vi "LaunchGUI.vi"(6 "Array":refnum<vi>[](array[refnum]), 10 "CtlRef":refnum<vi>, 11 "User Event in":refnum<user-event>) -> ()   [LabVIEW 2013]
uses:
  Controls/eventtypdef1.ctl
  Controls/controlFGV_TYPDEF.ctl
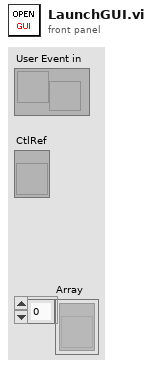
[diagram p1: front panel]
types:
  T1 = typedef "controlFGV_TYPDEF.ctl" = enum16{"read", "write", "clear"}
  T2 = typedef "eventtypdef1.ctl" = cluster{"label":string, "Sub Panel":refnum<vi>, "CtlRef":refnum<vi>, "This VI":refnum<vi>}
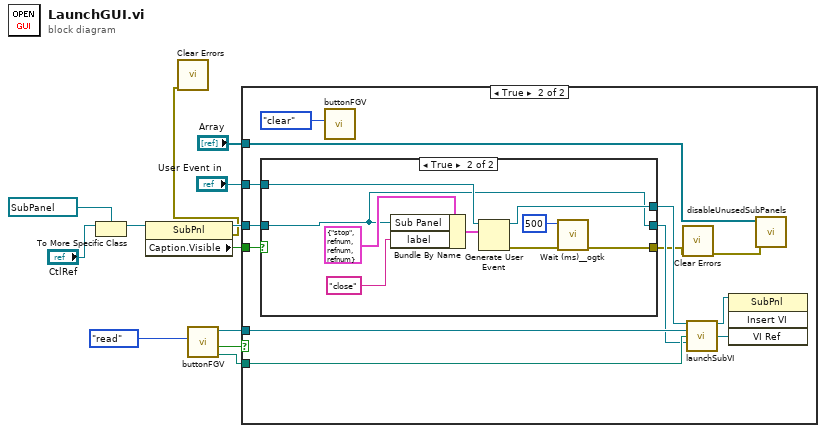
[diagram p0: block diagram]
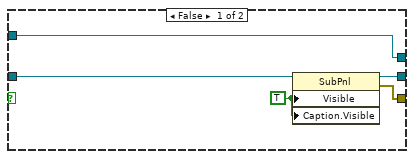
[diagram p3: hidden frame]
diagram:
  n1 = To More Specific Class(target class=refnum<vi> refnum ("Sub Panel"), reference="CtlRef") -> (specific class reference=w12:refnum<vi>)  [unwired: 1 in, 1 out]
  n2 = property class="SubPnl"(reference=w12) -> (reference out=w3:refnum<vi>, error out=w1:errorcluster, "Caption.Visible"=w8:bool)  [unwired: 1 in]
  n3 = call <vilib>:"Clear Errors.vi"("error in (no error)"=w1) -> ()  [unwired: 6 in, 1 out]
  n4 = call "buttonFGV.vi"("command"=controlFGV_TYPDEF."read") -> ("Path"=w6:path, "select subPanel"=w9:bool, "Boolean out"=w7:refnum<vi>)  [unwired: 8 in]
  n5 = case shown="True" w9 {
    tunnel: w6 -> [_ w25]
    tunnel: "User Event in" -> [_ w16]
    tunnel: w7 -> [_ w23]
    tunnel: "Array" -> [_ w24]
    tunnel: w8 -> [_ w17]
    tunnel: w3 -> [_ w22]
    frame False {
    }
    frame True {
      n6 = case shown="True" w17 {
        tunnel: [w29 w33] -> w14
        tunnel: w22 -> [w28 w36]
        tunnel: [w27 w36] -> w21
        tunnel: w16 -> [w26 w39]
        tunnel: [w26 w38] -> w15
        frame False {
          w30 = TRUE ("Visible")
          n7 = property class="SubPnl"(reference=w28, "Visible"=w30, "Caption.Visible"=w30) -> (reference out=w27:refnum<vi>, error out=w29:errorcluster)  [unwired: 1 in]
        }
        frame True {
          n8 = Bundle By Name(cluster=T2 {"label"="stop", "Sub Panel"=refnum, "CtlRef"=refnum, "This VI"=refnum} ("event data"), "Sub Panel"=w36, "label"="close") -> (w31:T2)
          n9 = Generate User Event(user event=w39, event data cluster=w31) -> (user event out=w38:refnum<user-event>, error out=w34:errorcluster)  [unwired: 2 in]
          n10 = call <userlib>:"Wait (ms)__ogtk.vi"("error in (no error)"=w34, "milliseconds to wait"=u32 500) -> ("error out"=w33:errorcluster)  [unwired: 8 in, 1 out]
        }
      }
      n11 = call "buttonFGV.vi"("command"=controlFGV_TYPDEF."clear") -> ()  [unwired: 8 in, 3 out]
      n12 = call <vilib>:"Clear Errors.vi"("error in (no error)"=w14) -> ("error out"=w13:errorcluster)  [unwired: 6 in]
      n13 = call "launchSubVI.vi"("User Event in"=w15, "Boolean out"=w23, "Path"=w25, "Sub Panel"=w21) -> ("Sub Panel out"=w20:refnum<vi>, "vi out"=w19:refnum<vi>)  [unwired: 10 in]
      n14 = invoke class="SubPnl" method="Insert VI"(reference=w20, "VI Ref"=w19) -> ()  [unwired: 2 in, 4 out]
      n15 = call "disableUnusedSubPanels.vi"("error in (no error)"=w13, "Array"=w24) -> ()  [unwired: 10 in]
    }
  }
